vi "save DSF Configuration to file.vi"(7 "prompt (Choose or enter file path)":string, 8 "error in (no error)":errorcluster, 10 "file (use dialog)":path, 11 "configuration cluster":T1) -> (0 "error out":errorcluster, 2 "path":path, 3 "configuration cluster out":T1)   [LabVIEW 2017, in "DSF Configuration API v1.0.0.lvlib"]
uses:
  DSF Configuration API v1.0.0.lvlib
  Controls/dsf configuration file/1.0.0/dsf configuration.ctl
  Controls/dsf configuration file/1.0.0/version.ctl
  Controls/dsf configuration file/1.0.0/dsf plugin.ctl
  Controls/dsf configuration file/1.0.0/dsf timing.ctl
  Controls/dsf configuration file/1.0.0/dsf group.ctl
  Controls/dsf configuration file/1.0.0/dsf transfer.ctl
  Controls/dsf configuration file/1.0.0/dsf channel.ctl
  Controls/dsf configuration file/1.0.0/dsf settings.ctl
  Controls/dsf configuration file/1.0.0/dsf configuration file v1.0.0.lvlib
panel:
  # "dsf\nfile"
  # "dsf\nfile"
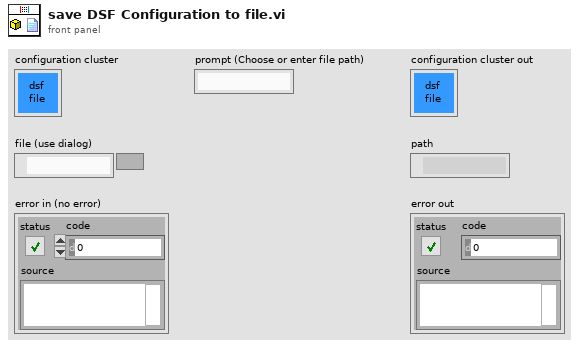
[diagram p1: front panel]
types:
  T1 = typedef "dsf configuration file v1.0.0.lvlib/dsf configuration.ctl" = cluster{"dsf":T2, "configuration":T2, "plugins":T3[], "groups":T5[], "transfers":T6[], "channels":T7[], "settings":T8[]}
  T2 = typedef "dsf configuration file v1.0.0.lvlib/version.ctl" = cluster{"major":u32, "minor":u32, "fix":u32, "build":string}
  T3 = typedef "dsf configuration file v1.0.0.lvlib/dsf plugin.ctl" = cluster{"id":string, "values":cluster{"type":string, "timing":T4, "group ids":string[], "settings id":string}}
  T4 = typedef "dsf configuration file v1.0.0.lvlib/dsf timing.ctl" = cluster{"decimation":i32, "offset":i32}
  T5 = typedef "dsf configuration file v1.0.0.lvlib/dsf group.ctl" = cluster{"id":string, "values":cluster{"direction":i32, "timing":T4, "transfer ids":string[], "settings id":string}}
  T6 = typedef "dsf configuration file v1.0.0.lvlib/dsf transfer.ctl" = cluster{"id":string, "values":cluster{"byte order":i32, "channel ids":string[], "settings id":string}}
  T7 = typedef "dsf configuration file v1.0.0.lvlib/dsf channel.ctl" = cluster{"id":string, "values":cluster{"count":i32, "offset":i32, "data type":i32, "resource path":string, "settings id":string}}
  T8 = typedef "dsf configuration file v1.0.0.lvlib/dsf settings.ctl" = cluster{"id":string, "values":cluster{"key":string, "value":string}[]}
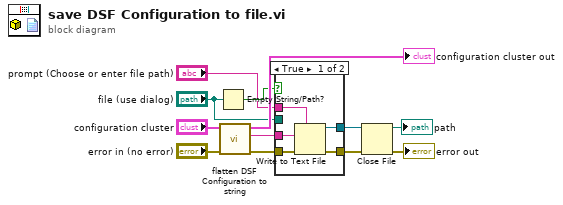
[diagram p0: block diagram]
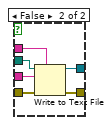
[diagram p2: hidden frame]
diagram:
  n1 = Empty String/Path?(string/path="file (use dialog)") -> (empty?=w3:bool)
  n2 = call "flatten DSF Configuration to string.vi"("error in (no error)"="error in (no error)", "configuration cluster in"="configuration cluster") -> ("error out"=w11:errorcluster, "string"=w10:string, "configuration cluster out"=→"configuration cluster out":T1)  [unwired: 7 in]
  n3 = case shown="True" w3 {
    tunnel: w11 -> [w17 w23]
    tunnel: w10 -> [w16 w22]
    tunnel: [w15 w21] -> w8
    tunnel: [w14 w20] -> w6
    tunnel: "file (use dialog)" -> [_ w18]
    tunnel: "prompt (Choose or enter file path)" -> [w13 w19]
    frame True {
      n4 = Write to Text File(prompt (Choose or enter file path)=w13, text=w16, error in=w17) -> (refnum out=w14:refnum<file>, error out=w15:errorcluster)  [unwired: 1 in, 1 out]
    }
    frame False {
      n5 = Write to Text File(prompt (Choose or enter file path)=w19, file (use dialog)=w18, text=w22, error in=w23) -> (refnum out=w20:refnum<file>, error out=w21:errorcluster)  [unwired: 1 out]
    }
  }
  n6 = Close File(refnum=w6, error in=w8) -> (path=→"path":path, error out=→"error out":errorcluster)
